vi "Read Cells.vi"(8 "error in (no error)":errorcluster, 11 "CRDS in":refnum<class "CRDS.lvclass">) -> (0 "error out":errorcluster, 2 "Cells":refnum<class "CRDS Cell.lvclass">[](array[class]), 3 "CRDS out":refnum<class "CRDS.lvclass">)   [LabVIEW 2015, in "CRDS Lib.lvlib" / "CRDS.lvclass"]
uses:
  CRDS.lvclass
  Cell/CRDS Cell.lvclass
  CRDS.lvclass/CRDS.ctl
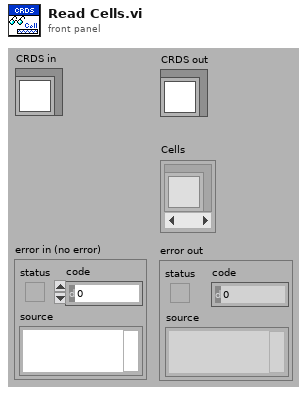
[diagram p1: front panel]
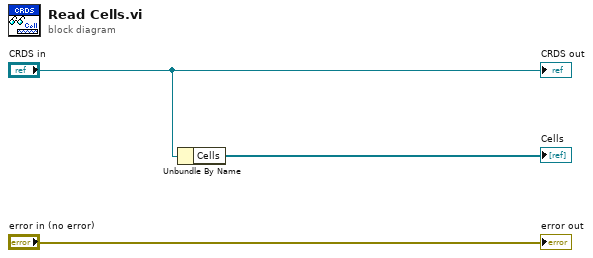
[diagram p0: block diagram]
diagram:
  n1 = Unbundle By Name("CRDS in") -> ("Cells"=→"Cells":refnum<class "CRDS Cell.lvclass">[])
  "error out" <- "error in (no error)"
  "CRDS out" <- "CRDS in"
